vi "rad_Compare Software.vi"(8 "Installed Software 2":string[](array[string]), 11 "Installed Software 1":string[](array[string])) -> (0 "Analyzed Software 2":T1(array[cluster]), 1 "Different version":i32, 2 "Same version":i32, 3 "Analyzed Software 1":T1(array[cluster]))   [LabVIEW 2016]
panel:
  in  "Installed Component":T2
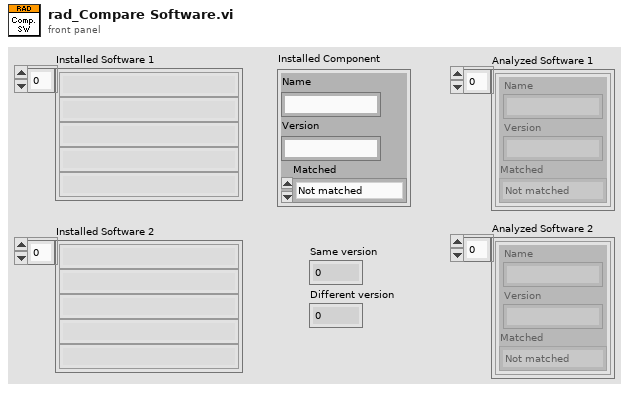
[diagram p1: front panel]
types:
  T1 = cluster{"Name":string, "Version":string, "Matched":enum16{"Not matched", "Different version", "Same version"}}[]
  T2 = cluster{"Name":string, "Version":string, "Matched":enum16{"Not matched", "Different version", "Same version"}}
  T3 = enum16{"Not matched", "Different version", "Same version"}
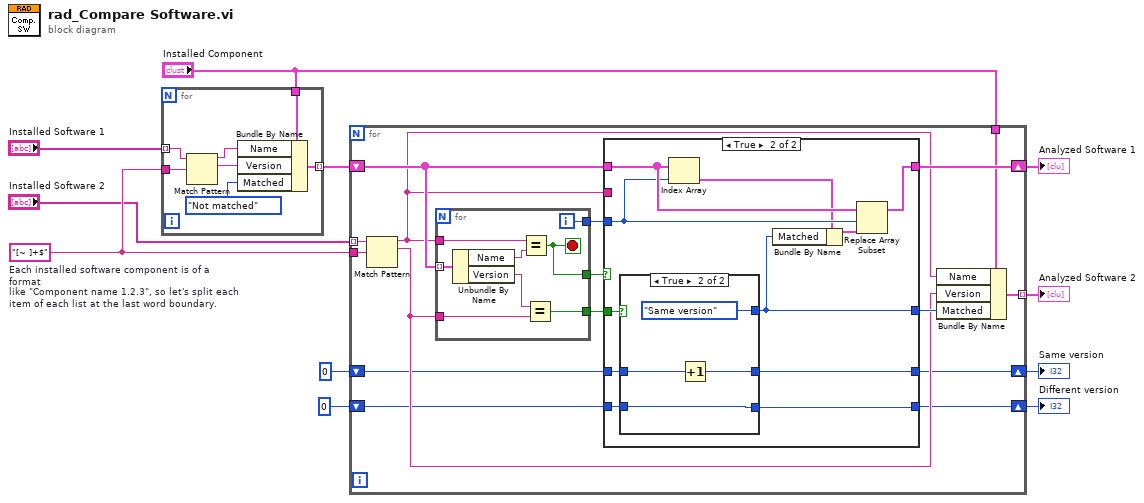
[diagram p0: block diagram]
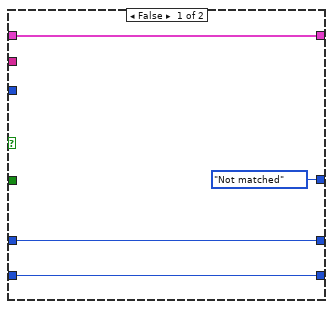
[diagram p2: hidden frame]
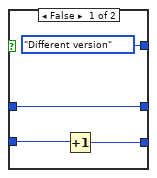
[diagram p3: hidden frame]
diagram:
  w10 = "[~ ]+$"  # Each installed software component is of a format like "Component name 1.2.3", so let's split each item of each list at the last word boundary.
  n1 = for {
    tunnel: "Installed Software 1" -> [w18] mode=indexing
    tunnel: [w15] -> w8 mode=indexing
    tunnel: "Installed Component" -> [w14]
    tunnel: w10 -> [w13]
    n2 = Match Pattern(string=w18, regular expression=w13) -> (before substring=w17:string, match substring=w16:string)  [unwired: 1 in, 2 out]
    n3 = Bundle By Name(cluster=w14, "Name"=w17, "Version"=w16, "Matched"=T3."Not matched") -> (w15:T2)
  }
  n4 = for {
    shift-right: [w32] -> w2
    shift-left: w8 -> [w31]
    tunnel: "Installed Software 2" -> [w34] mode=indexing
    tunnel: "Installed Component" -> [w27]
    tunnel: w10 -> [w29]
    tunnel: [w26] -> w1 mode=indexing
    shift-right: [w21] -> w5
    shift-left: 0 ("Same version") -> [w22]
    shift-right: [w19] -> w4
    shift-left: 0 ("Different version") -> [w20]
    n5 = Match Pattern(string=w34, regular expression=w29) -> (before substring=w25:string, match substring=w24:string)  [unwired: 1 in, 2 out]
    n6 = for {
      tunnel: w31 -> [w65] mode=indexing
      tunnel: w25 -> [w62]
      tunnel: [w64] -> w30
      tunnel: [w63] -> w33
      tunnel: w24 -> [w59]
      tunnel: [w58] -> w23
      i -> [w64]
      stop <- w63 stop-if-true
      n7 = Unbundle By Name(w65) -> ("Name"=w61:string, "Version"=w60:string)
      n8 = Equal?(x=w62, y=w61) -> (x = y?=w63:bool)
      n9 = Equal?(x=w60, y=w59) -> (x = y?=w58:bool)
    }
    n10 = case shown="True" w33 {
      tunnel: [w38 w45] -> w32
      tunnel: w31 -> [w38 w49]
      tunnel: w25 -> [_ _]
      tunnel: w30 -> [_ w48]
      tunnel: [T3."Not matched" ("Matched") w43] -> w28
      tunnel: w23 -> [_ w44]
      tunnel: w22 -> [w36 w39]
      tunnel: [w36 w40] -> w21
      tunnel: w20 -> [w35 w42]
      tunnel: [w35 w41] -> w19
      frame False {
      }
      frame True {
        n11 = case shown="True" w44 {
          tunnel: [T3."Different version" T3."Same version"] -> w43
          tunnel: w42 -> [w52 w54]
          tunnel: [w51 w54] -> w41
          tunnel: [w50 w55] -> w40
          tunnel: w39 -> [w50 w56]
          frame False {
            n12 = Increment(x=w52) -> (x+1=w51:i32)
          }
          frame True {
            n13 = Increment(x=w56) -> (x+1=w55:i32)
          }
        }
        n14 = Index Array(array=w49, index=w48) -> (element=w47:T2)
        n15 = Bundle By Name(cluster=w47, "Matched"=w43) -> (w46:T2)
        n16 = Replace Array Subset(array=w49, new element=w46, index=w48) -> (w45:T1)
      }
    }
    n17 = Bundle By Name(cluster=w27, "Name"=w25, "Version"=w24, "Matched"=w28) -> (w26:T2)
  }
  "Same version" <- w5
  "Different version" <- w4
  "Analyzed Software 1" <- w2
  "Analyzed Software 2" <- w1
